vi "Check if In LabVIEW Dir.vi"(2 "VI Refnum":refnum<vi>) -> (0 "Boolean":bool)   [LabVIEW 2017, in "csm-ui-support.lvlib"]
uses:
  csm-ui-support.lvlib
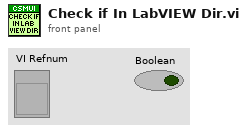
[diagram p1: front panel]
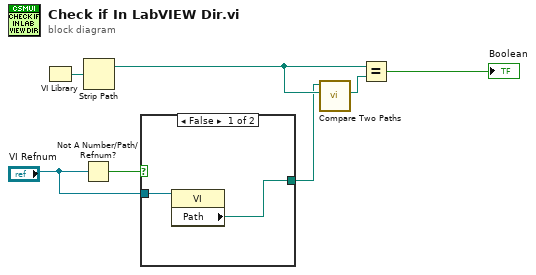
[diagram p0: block diagram]
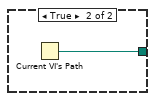
[diagram p2: hidden frame]
diagram:
  n1 = VI Library() -> (path=w3:path)
  n2 = Not A Number/Path/Refnum?(number/path/refnum="VI Refnum") -> (NaN/Path/Refnum?=w2:bool)
  n3 = Strip Path(path=w3) -> (stripped path=w6:path)  [unwired: 1 out]
  n4 = case shown="False" w2 {
    tunnel: [w8 w10] -> w4
    tunnel: "VI Refnum" -> [w9 _]
    frame False {
      n5 = property class="VI"(reference=w9) -> ("Path"=w8:path)  [unwired: 1 in, 2 out]
    }
    frame True {
      n6 = Current VI's Path() -> (path=w10:path)
    }
  }
  n7 = call <vilib>:"Compare Two Paths.vi"("Path 2"=w6, "Path 1"=w4) -> ("Common Path"=w5:path)  [unwired: 6 in, 3 out]
  n8 = Equal?(x=w6, y=w5) -> (x = y?=→"Boolean":bool)
